vi "RectAndRect.vi"(1 "rect b":T1, 2 "rect a":T1) -> (0 "union rect":T1)   [LabVIEW 2011]
panel:
  # "Union of two rects"
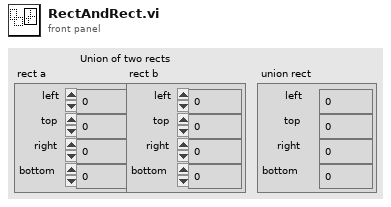
[diagram p1: front panel]
types:
  T1 = cluster{"left":i16, "top":i16, "right":i16, "bottom":i16}
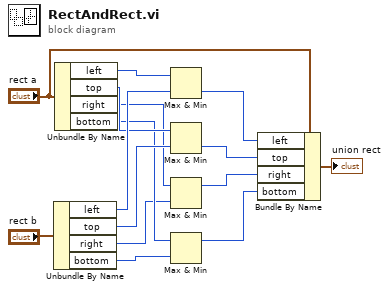
[diagram p0: block diagram]
diagram:
  n1 = Unbundle By Name("rect b") -> ("left"=w11:i16, "top"=w9:i16, "right"=w5:i16, "bottom"=w6:i16)
  n2 = Unbundle By Name("rect a") -> ("left"=w12:i16, "top"=w10:i16, "right"=w8:i16, "bottom"=w7:i16)
  n3 = Max & Min(x=w12, y=w11) -> (min(x,y)=w4:i16)  [unwired: 1 out]
  n4 = Max & Min(x=w10, y=w9) -> (min(x,y)=w3:i16)  [unwired: 1 out]
  n5 = Max & Min(x=w8, y=w5) -> (max(x,y)=w2:i16)  [unwired: 1 out]
  n6 = Max & Min(x=w7, y=w6) -> (max(x,y)=w1:i16)  [unwired: 1 out]
  n7 = Bundle By Name(cluster="rect a", "left"=w4, "top"=w3, "right"=w2, "bottom"=w1) -> (→"union rect":T1)
